vi "SECS Bridge Main.vi"() -> ()   [LabVIEW 2020, in "SECS Bridge.lvlib"]
uses:
  SECS Bridge.lvlib
  SECS Communication/HSMS Class/HSMS State.ctl
  SubVI/File FGV Method.ctl
  SubVI/Configuration.ctl
  SECS Communication/S7 Message Class/S7F4.ctl
  SECS Communication/S1 Message Class/S1F18.ctl
  SECS Communication/S2 Message Class/S2F32.ctl
  SECS Communication/HSMS Class/Notifier Data.ctl
  SECS Communication/HSMS Class/Notifier Type.ctl
  SECS Communication/SECS Data Class/Get ALID Data.vi
  SECS Communication/SECS Data Class/Put ALID Data.vi
  SECS Communication/HSMS Class/HSMS Class.lvclass
  SECS Scenarios/Scenarios Class/Scenarios Class.lvclass
  SECS Communication/SECS Data Class/SECS Data Class.lvclass
  SECS Communication/S7 Message Class/S7 Message Class.lvclass
  SECS Communication/S1 Message Class/S1 Message Class.lvclass
  SECS Communication/S2 Message Class/S2 Message Class.lvclass
panel:
  in  "Clear":bool
  in  "Stop":bool
  in  "Log View":bool
  in  "Configuration":bool
  in  "Stop SECS":bool
  in  "Start SECS":bool
  out "Version":string
  out "On-Line":bool
  in  "Notifier Data":i32(listbox)
  out "HSMS State":T1=enum."Stop"
  in  "Test Tab":enum32{"Broadcast Test", "Request Test"}(tab)
  in  "Enable Broadcast":bool
  out "PP-SELECT":string
  out "Set Equip. Time":string
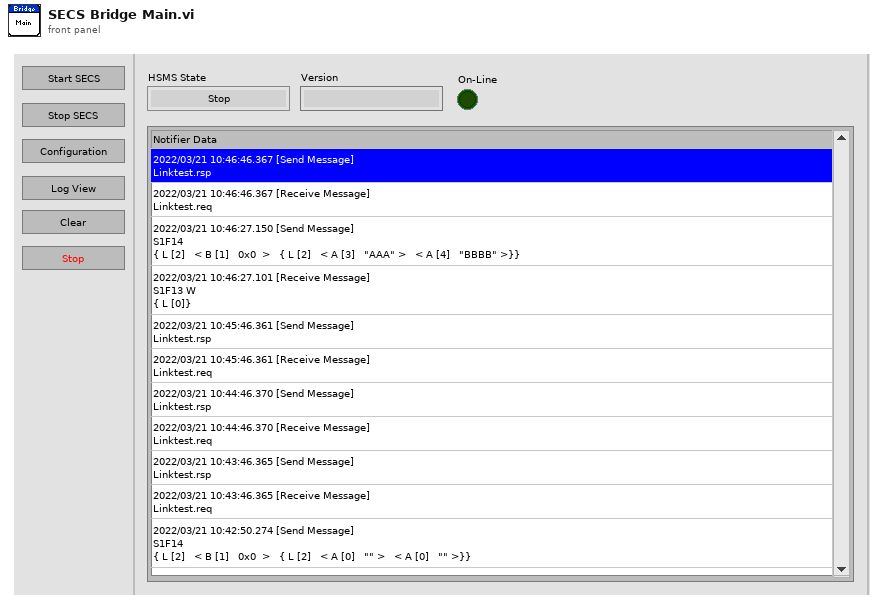
[diagram p1: front panel]
types:
  T1 = typedef "SECS Communication.lvlib/HSMS Class.lvclass/HSMS State.ctl" = enum16{"[TCP/IP]Not Connect", "[HSMS]Not Selected", "[HSMS]Selected", "Stop"}
  T2 = typedef "SECS Bridge.lvlib/Main Data Buffer.ctl" = cluster{"HSMS Class":refnum<class "HSMS Class.lvclass">, "SECS Data Class":refnum<class "SECS Data Class.lvclass">, "Scenarios Class":refnum<class "Scenarios Class.lvclass">, "VI Refnum":refnum<vi>, "Ctl Refnum Map":map{string, refnum<vi>}, "Timeout":i32, "Notifier Data":string[], "Event Refnum":refnum<event-registration>}
  T3 = enum16{"Null", "Normal", "Abnormal", "Warning", "Disable"}
  T4 = typedef "SECS Bridge.lvlib/File FGV Method.ctl" = enum16{"Get", "Put", "Read", "Write"}
  T5 = typedef "SECS Communication.lvlib/S7 Message Class.lvclass/S7F4.ctl" = enum8{"Accepted", "Permission not granted", "length error", "matrix overflow", "PPID not found", "unsupported mode", "initiated for asynchronous completion", "storage limit error"}
  T6 = typedef "SECS Bridge.lvlib/Configuration.ctl" = cluster{"T3(Reply Timeout)":i32, "T5(Separation Timeout)":i32, "T6(Control Timeout)":i32, "T7(Not Selected Timeout)":i32, "T8(Inter-Character Timeout)":i32, "Session ID":u16, "Log Path":path, "IP Address":string, "Port":u16}
  T7 = typedef "SECS Communication.lvlib/S1 Message Class.lvclass/S1F18.ctl" = enum16{"ok", "refused", "already online"}
  T8 = enum8{"ok, completed", "invalid command", "cannot do now", "parameter error", "initiated for asynchronous completion", "rejected, already in desired condition", "invalid object"}
  T9 = typedef "SECS Communication.lvlib/S2 Message Class.lvclass/S2F32.ctl" = enum16{"ok", "not done"}
  T10 = typedef "SECS Communication.lvlib/HSMS Class.lvclass/Notifier Data.ctl" = cluster{"Notifier Type":T11, "Data":variant, "Time":timestamp}
  T11 = typedef "SECS Communication.lvlib/HSMS Class.lvclass/Notifier Type.ctl" = enum16{"TCPIP Connect", "TCPIP Disconnect", "Receive Message", "Send Message", "T3 Timeout", "T6 Timeout", "T7 Timeout", "Error", "Stop"}
  T12 = typedef "SECS Scenarios.lvlib/Scenarios Class.lvclass/Broadcast Refnum.ctl" = cluster{"13-EnableDisable Alarm":refnum<user-event>, "15-Process Program Request":refnum<user-event>, "16-Process Program Send":refnum<user-event>, "17-Deleting a Process Program by Host":refnum<user-event>, "18-Host Requests Equipment Process Program Directory":refnum<user-event>, "19-Equipment Process Program Uploading":refnum<user-event>, "20[1]-Process Program Downloading":refnum<user-event>, "20[2]-Process Program Downloading":refnum<user-event>, "22-Host Sends Information to Equipment":refnum<user-event>, "26-Host Requests to Enter OFF-Line":refnum<user-event>, "27-Host Requests to Enter On-Line":refnum<user-event>, "28[1]-Remote Control[PP-SELECT]":refnum<user-event>, "28[2]-Remote Control[START]":refnum<user-event>, "28[3]-Remote Control[STOP]":refnum<user-event>, "28[4]-Remote Control[LOCAL]":refnum<user-event>, "28[5]-Remote Control[REMOTE]":refnum<user-event>, "28[6]-Remote Control[RCMD]":refnum<user-event>, "30-Host Requests Equipment to Set Time":refnum<user-event>, "31-Host Requests Time Value from Equipment":refnum<user-event>, "32[1]-Trace Data Collection":refnum<user-event>, "32[2]-Trace Data Collection":refnum<user-event>}
  T13 = typedef "SECS Communication.lvlib/SECS Data Class.lvclass/ALID Data.ctl" = cluster{"Enable":bool, "ALID":u32, "Name":string, "Description":string, "Source":string, "Status":enum16{"Null", "Normal", "Abnormal", "Warning"}}
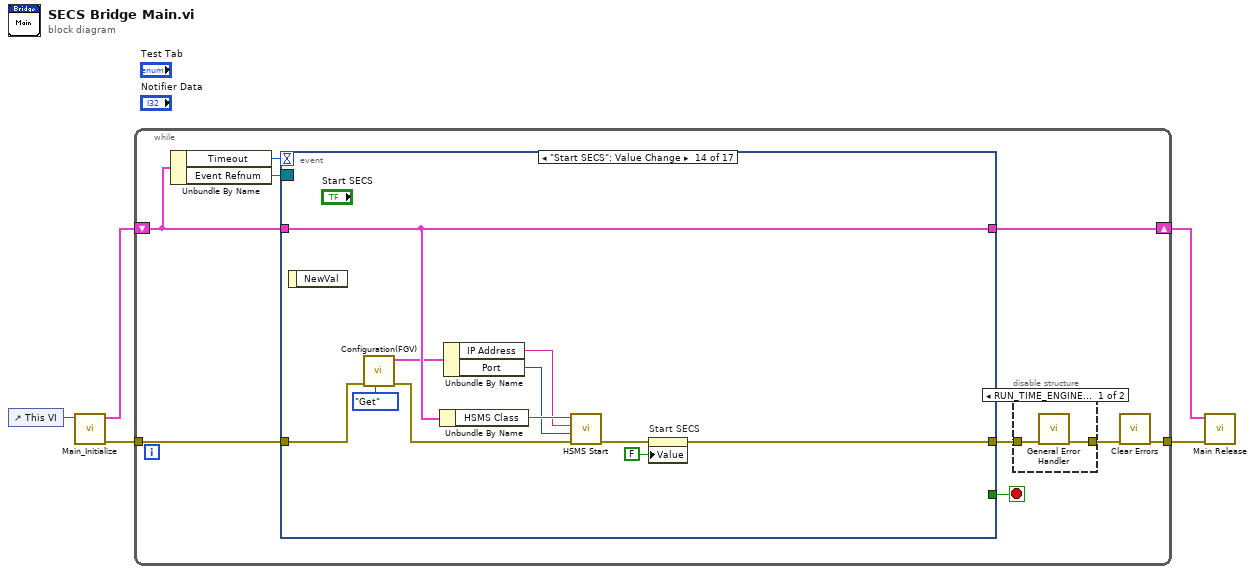
[diagram p0: block diagram]
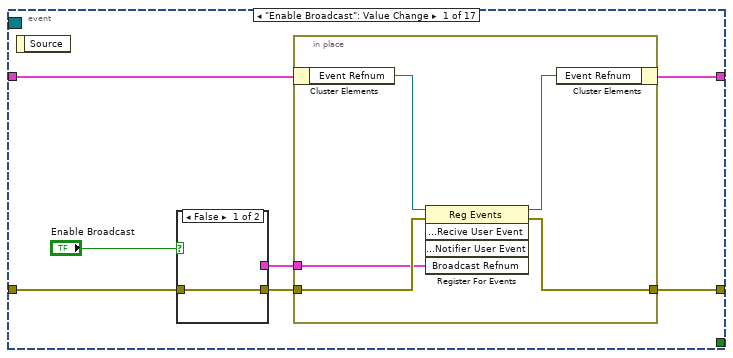
[diagram p3: hidden frame]
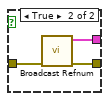
[diagram p4: hidden frame]
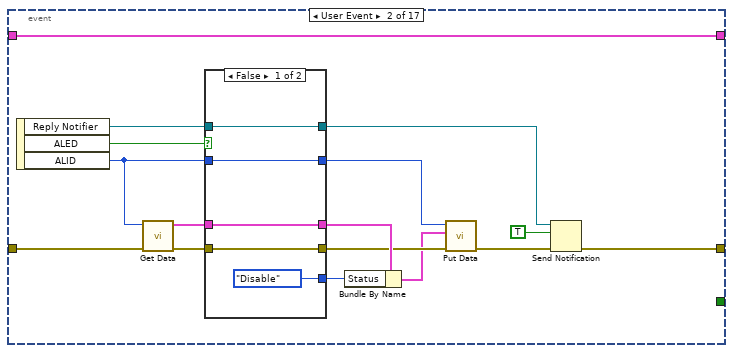
[diagram p5: hidden frame]
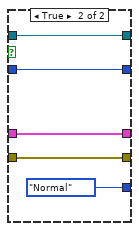
[diagram p6: hidden frame]
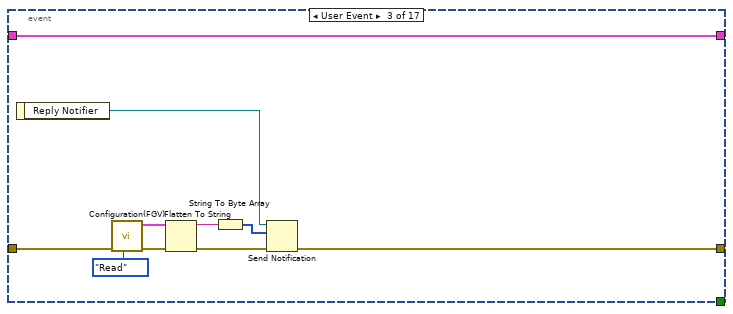
[diagram p7: hidden frame]
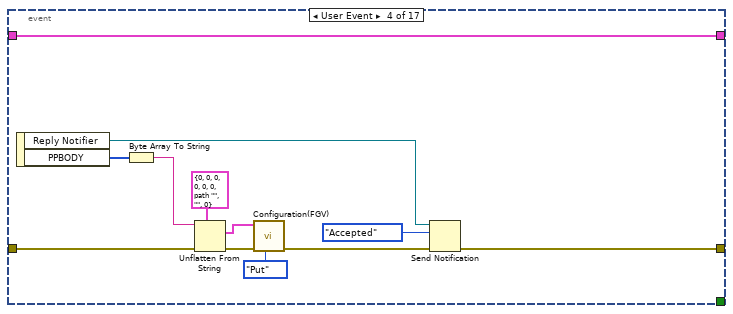
[diagram p8: hidden frame]
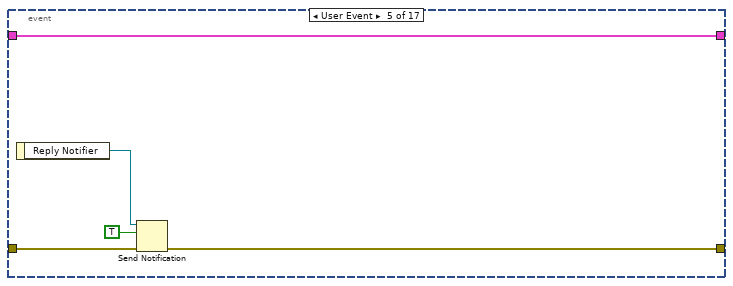
[diagram p9: hidden frame]
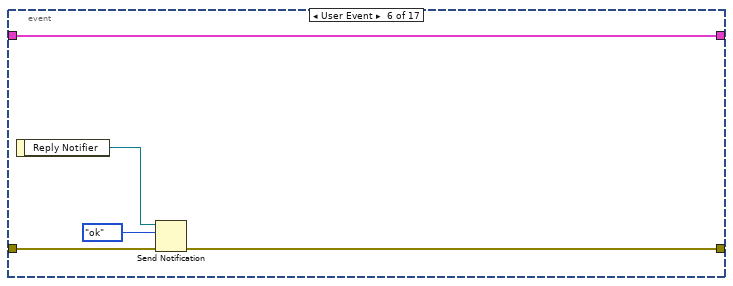
[diagram p10: hidden frame]
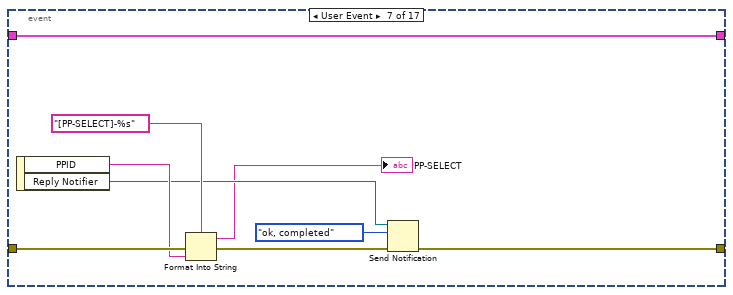
[diagram p11: hidden frame]
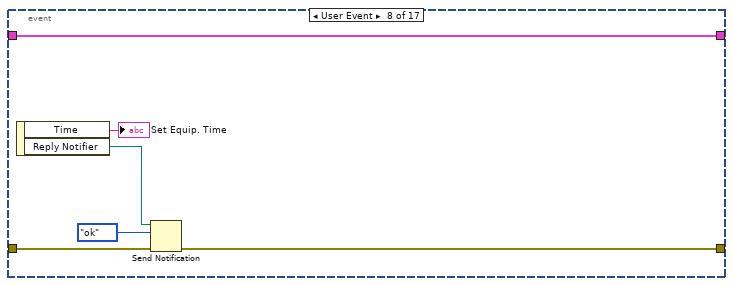
[diagram p12: hidden frame]
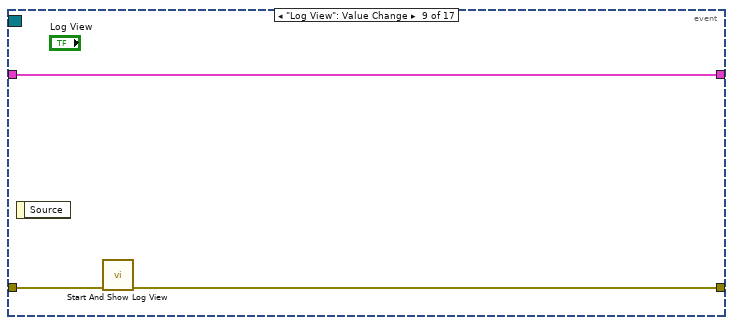
[diagram p13: hidden frame]
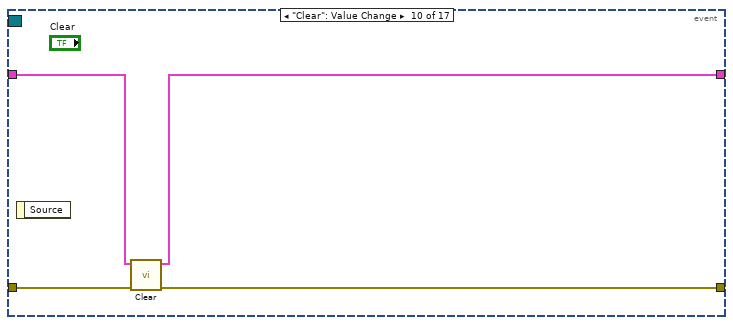
[diagram p14: hidden frame]
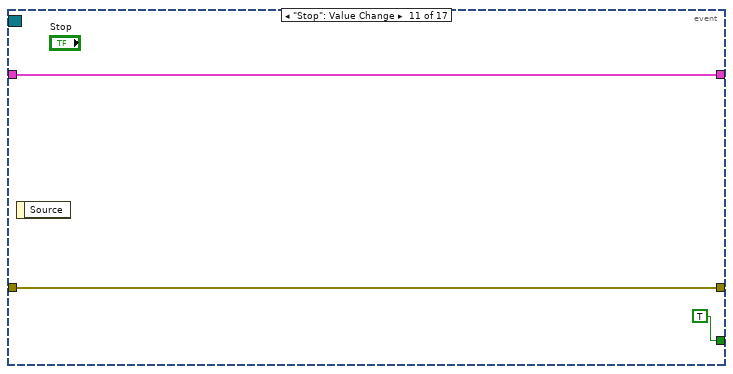
[diagram p15: hidden frame]
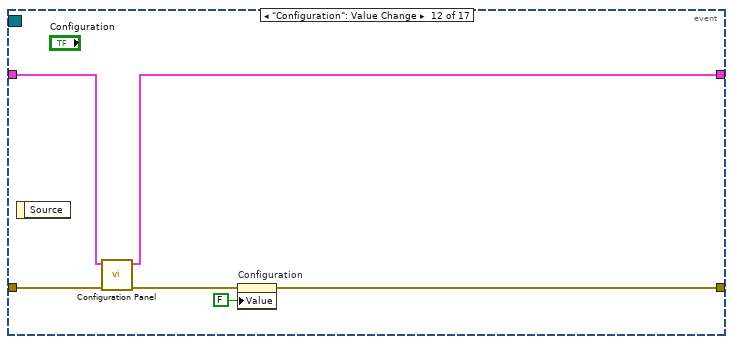
[diagram p16: hidden frame]
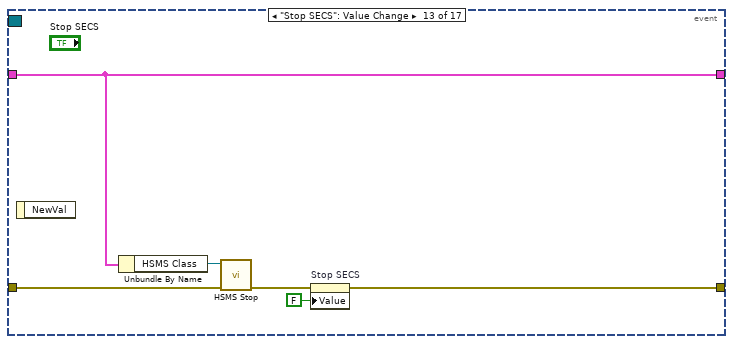
[diagram p17: hidden frame]
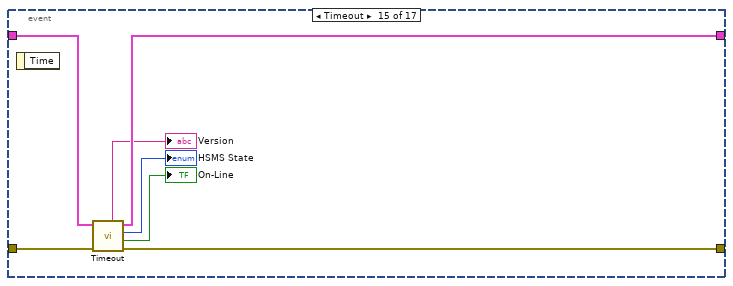
[diagram p18: hidden frame]
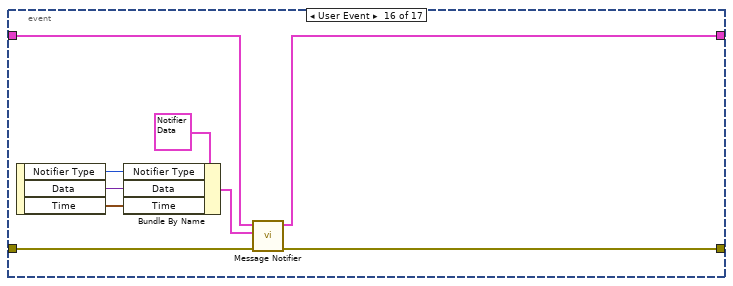
[diagram p19: hidden frame]
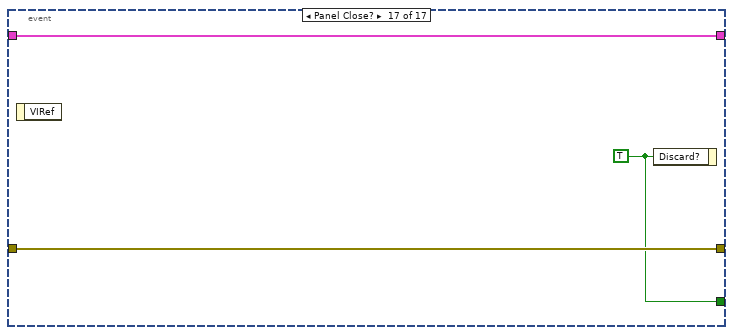
[diagram p20: hidden frame]
diagram:
  n1 = control-ref of="This VI"() -> (w5:refnum<vi>)
  n2 = call "Main_Initialize.vi"("VI Refnum"=w5) -> ("error out"=w1:errorcluster, "Main Data Buffer"=w2:T2)  [unwired: 9 in]
  n3 = while {
    tunnel: w1 -> [w11]
    shift-right: [w10] -> w3
    shift-left: w2 -> [w12]
    tunnel: [w6] -> w4
    stop <- w9 stop-if-true
    n4 = Unbundle By Name(w12) -> ("Timeout"=w14:i32, "Event Refnum"=w13:refnum<event-registration>)
    n5 = event shown="[13] \"Start SECS\": Value Change" {
      selector: w13 -> [_ _ _ _ _ _ _ _ _ _ _ _ _ _ _ _ _]
      dyn-events: _ -> [_ _ _ _ _ _ _ _ _ _ _ _ _ _ _ _ _]
      timeout: w14 -> [_ _ _ _ _ _ _ _ _ _ _ _ _ _ _ _ _]
      tunnel: w12 -> [w22 w36 w69 w72 w86 w91 w99 w104 w109 w112 w116 w121 w126 w139 w145 w149 w158]
      tunnel: w11 -> [w24 w49 w66 w81 w85 w90 w100 w106 w108 w113 w115 w122 w128 w137 w146 w151 w157]
      tunnel: [w18 w36 w69 w72 w86 w91 w99 w104 w109 w111 w116 w120 w126 w139 w144 w148 w158] -> w10
      tunnel: [w19 w35 w60 w71 w82 w87 w94 w103 w107 w110 w115 w118 w124 w130 w143 w147 w157] -> w8
      tunnel: [_ _ _ _ _ _ _ _ _ _ TRUE ("Discard?") _ _ _ _ _ w156] -> w9
      event "Enable Broadcast": Value Change {
        n6 = event-data() -> ()  [unwired: 1 in, 1 out]
        n7 = case shown="False" "Enable Broadcast" {
          tunnel: w24 -> [w30 w33]
          tunnel: [w30 w32] -> w21
          tunnel: [_ w31] -> w20
          frame False {
          }
          frame True {
            n8 = call "Broadcast Refnum.vi"("error in"=w33) -> ("error out"=w32:errorcluster, "Broadcast Refnum"=w31:T12)  [unwired: 9 in]
          }
        }
        n9 = in-place {
          in-place-border: w21 -> [w29]
          in-place-border: w20 -> [w27]
          in-place-border: [w25] -> w19
          n10 = in-place-cluster #1(w22) -> ("Event Refnum"=w28:refnum<event-registration>)
          n11 = register-events(reference=w28, error in=w29, w27) -> (reference out=w26:refnum<event-registration>, error out=w25:errorcluster)  [unwired: 2 in]
          n12 = in-place-cluster #1("Event Refnum"=w26) -> (w18:T2)
        }
      }
      event User Event {
        n13 = event-data() -> ("Reply Notifier"=w39:refnum<notifier>, "ALED"=w47:bool, "ALID"=w41:u32)  [unwired: 1 in]
        n14 = call-poly "Get Data.vi"("error in"=w49, "ALID"=w41) -> ("error out"=w48:errorcluster, "ALID Data"=w46:T13)  [unwired: 7 in, 1 out]
        n15 = case shown="False" w47 {
          tunnel: w48 -> [w53 w58]
          tunnel: w46 -> [w54 w59]
          tunnel: [w54 w59] -> w45
          tunnel: [w53 w58] -> w43
          tunnel: [T3."Disable" ("Status") T3."Normal" ("Status")] -> w44
          tunnel: w41 -> [w51 w56]
          tunnel: [w51 w56] -> w40
          tunnel: w39 -> [w50 w55]
          tunnel: [w50 w55] -> w37
          frame False {
          }
          frame True {
          }
        }
        n16 = Bundle By Name(cluster=w45, "Status"=w44) -> (w42:T13)
        n17 = call-poly "Put Data.vi"("error in"=w43, "ALID Data"=w42, "ALID"=w40) -> ("error out"=w38:errorcluster)  [unwired: 7 in, 1 out]
        n18 = Send Notification(notification=TRUE, notifier=w37, error in (no error)=w38) -> (error out=w35:errorcluster)  [unwired: 1 out]
      }
      event User Event {
        n19 = event-data() -> ("Reply Notifier"=w68:refnum<notifier>)  [unwired: 1 in]
        n20 = call "Configuration(FGV).vi"("File FGV Method"=File_FGV_Method."Read", "error in"=w66) -> ("error out"=w65:errorcluster, "Configuration Out"=w64:T6)  [unwired: 8 in]
        n21 = Flatten To String(anything=w64, error in (no error)=w65) -> (data string=w63:string, error out=w62:errorcluster)  [unwired: 2 in, 1 out]
        n22 = String To Byte Array(string=w63) -> (unsigned byte array=w61:u8[])
        n23 = Send Notification(notification=w61, notifier=w68, error in (no error)=w62) -> (error out=w60:errorcluster)  [unwired: 1 out]
      }
      event User Event {
        n24 = event-data() -> ("Reply Notifier"=w73:refnum<notifier>, "PPBODY"=w80:u8[])  [unwired: 1 in]
        n25 = Byte Array To String(unsigned byte array=w80) -> (string=w79:string)
        n26 = Unflatten From String(type=T6 {"T3(Reply Timeout)"=0, "T5(Separation Timeout)"=0, "T6(Control Timeout)"=0, "T7(Not Selected Timeout)"=0, "T8(Inter-Character Timeout)"=0, "Session ID"=0, "Log Path"=path "", "IP Address"="", "Port"=0} ("Configuration In"), binary string=w79, error in (no error)=w81) -> (value=w75:T6, error out=w78:errorcluster)  [unwired: 2 in, 1 out]
        n27 = call "Configuration(FGV).vi"("File FGV Method"=File_FGV_Method."Put", "error in"=w78, "Configuration In"=w75) -> ("error out"=w74:errorcluster)  [unwired: 7 in, 1 out]
        n28 = Send Notification(notification=S7F4."Accepted", notifier=w73, error in (no error)=w74) -> (error out=w71:errorcluster)  [unwired: 1 out]
      }
      event User Event {
        n29 = event-data() -> ("Reply Notifier"=w84:refnum<notifier>)  [unwired: 1 in]
        n30 = Send Notification(notification=TRUE, notifier=w84, error in (no error)=w85) -> (error out=w82:errorcluster)  [unwired: 1 out]
      }
      event User Event {
        n31 = event-data() -> ("Reply Notifier"=w89:refnum<notifier>)  [unwired: 1 in]
        n32 = Send Notification(notification=S1F18."ok", notifier=w89, error in (no error)=w90) -> (error out=w87:errorcluster)  [unwired: 1 out]
      }
      event User Event {
        n33 = event-data() -> ("PPID"=w98:string, "Reply Notifier"=w95:refnum<notifier>)  [unwired: 1 in]
        n34 = Format Into String(format string="[PP-SELECT]-%s", error in=w100, w98) -> (resulting string=→"PP-SELECT":string, error out=w96:errorcluster)  [unwired: 1 in]
        n35 = Send Notification(notification=T8."ok, completed", notifier=w95, error in (no error)=w96) -> (error out=w94:errorcluster)  [unwired: 1 out]
      }
      event User Event {
        n36 = event-data() -> ("Time"=→"Set Equip. Time":string, "Reply Notifier"=w105:refnum<notifier>)  [unwired: 1 in]
        n37 = Send Notification(notification=S2F32."ok", notifier=w105, error in (no error)=w106) -> (error out=w103:errorcluster)  [unwired: 1 out]
      }
      event "Log View": Value Change {
        n38 = event-data() -> ()  [unwired: 1 in, 1 out]
        n39 = call "Start And Show Log View.vi"("error in"=w108) -> ("error out"=w107:errorcluster)  [unwired: 10 in]
      }
      event "Clear": Value Change {
        n40 = event-data() -> ()  [unwired: 1 in, 1 out]
        n41 = call "Clear.vi"("error in"=w113, "Main Data Buffer In"=w112) -> ("error out"=w110:errorcluster, "Main Data Buffer Out"=w111:T2)  [unwired: 8 in]
      }
      event "Stop": Value Change {
        n42 = event-data() -> ()  [unwired: 1 in, 1 out]
      }
      event "Configuration": Value Change {
        n43 = event-data() -> ()  [unwired: 1 in, 1 out]
        n44 = call "Configuration Panel.vi"("error in"=w122, "Main Data Buffer In"=w121) -> ("error out"=w119:errorcluster, "Main Data Buffer Out"=w120:T2)  [unwired: 8 in]
        n45 = property on="Configuration" class="Bool (strict)"(error in=w119, "Value"=FALSE ("Configuration")) -> (error out=w118:errorcluster)  [unwired: 1 in, 1 out]
      }
      event "Stop SECS": Value Change {
        n46 = event-data() -> ()  [unwired: 1 in, 1 out]
        n47 = Unbundle By Name(w126) -> ("HSMS Class"=w127:refnum<class "HSMS Class.lvclass">)
        n48 = call "HSMS Stop.vi"("error in (no error)"=w128, "HSMS Class in"=w127) -> ("error out"=w125:errorcluster)  [unwired: 8 in, 1 out]
        n49 = property on="Stop SECS" class="Bool (strict)"(error in=w125, "Value"=FALSE ("Stop SECS")) -> (error out=w124:errorcluster)  [unwired: 1 in, 1 out]
      }
      event "Start SECS": Value Change {
        n50 = event-data() -> ()  [unwired: 1 in, 1 out]
        n51 = call "Configuration(FGV).vi"("File FGV Method"=File_FGV_Method."Get", "error in"=w137) -> ("error out"=w136:errorcluster, "Configuration Out"=w135:T6)  [unwired: 8 in]
        n52 = Unbundle By Name(w139) -> ("HSMS Class"=w138:refnum<class "HSMS Class.lvclass">)
        n53 = Unbundle By Name(w135) -> ("IP Address"=w132:string, "Port"=w133:u16)
        n54 = call "HSMS Start.vi"("error in (no error)"=w136, "Port"=w133, "IP Adrress"=w132, "HSMS Class in"=w138) -> ("error out"=w131:errorcluster)  [unwired: 6 in, 1 out]
        n55 = property on="Start SECS" class="Bool (strict)"(error in=w131, "Value"=FALSE ("Start SECS")) -> (error out=w130:errorcluster)  [unwired: 1 in, 1 out]
      }
      event Timeout {
        n56 = event-data() -> ()  [unwired: 1 in, 1 out]
        n57 = call "Timeout.vi"("error in"=w146, "Main Data Buffer In"=w145) -> ("error out"=w143:errorcluster, "On-Line"=→"On-Line":bool, "HSMS State"=→"HSMS State":T1, "Main Data Buffer Out"=w144:T2, "Version"=→"Version":string)  [unwired: 5 in]
      }
      event User Event {
        n58 = event-data() -> ("Notifier Type"=w152:T11, "Data"=w153:variant, "Time"=w154:timestamp)  [unwired: 1 in]
        n59 = Bundle By Name(cluster=T10 {"Notifier Type"=enum."Receive Message", "Data"=variant, "Time"=timestamp(0 s since 1904-01-01)} ("Notifier Data"), "Notifier Type"=w152, "Data"=w153, "Time"=w154) -> (w150:T10)
        n60 = call "Message Notifier.vi"("error in"=w151, "Notifier Data"=w150, "Main Data Buffer In"=w149) -> ("error out"=w147:errorcluster, "Main Data Buffer Out"=w148:T2)  [unwired: 7 in]
      }
      event Panel Close? {
        w156 = TRUE ("Discard?")
        n61 = event-data() -> ()  [unwired: 1 in, 1 out]
        n62 = event-data("Discard?"=w156) -> ()  [unwired: 1 in, 1 out]
      }
    }
    n63 = disable-structure shown="RUN_TIME_ENGINE==False, Default" {
      disable-tunnel: w8 -> [w16 w17]
      disable-tunnel: [w15 w17] -> w7
      frame condition #0 (active) {
        n64 = call <vilib>:"General Error Handler.vi"("error in (no error)"=w16) -> ("error out"=w15:errorcluster)  [unwired: 10 in, 4 out]
      }
      frame condition #1 {
      }
    }
    n65 = call <vilib>:"Clear Errors.vi"("error in (no error)"=w7) -> ("error out"=w6:errorcluster)  [unwired: 5 in, 1 out]
  }
  n66 = call "Main Release.vi"("error in"=w4, "Main Data Buffer"=w3) -> ()  [unwired: 9 in, 1 out]
